vi "Vision Center Shoot.vi"(0 "Intake":dbl=1.0, 1 "X axis value":dbl=0.05 format="%#_13g", 2 "X axis value 2":dbl=-0.05) -> ()   [LabVIEW 2015]
uses:
  Robot Global Data.vi
panel:
  in  "X axis value 3":dbl=0.05 format="%#_13g"
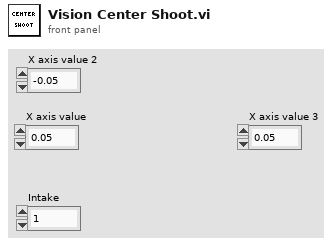
[diagram p1: front panel]
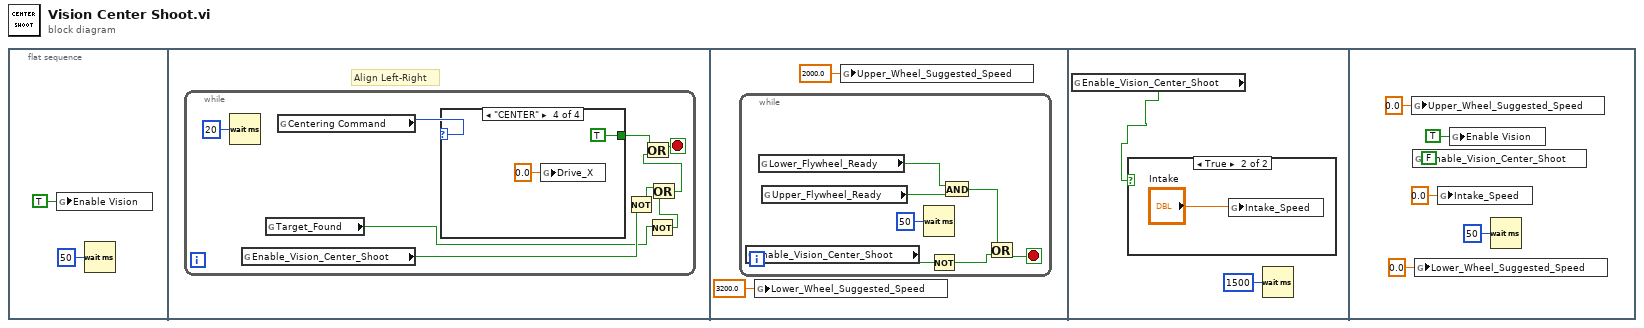
[diagram p0: block diagram]
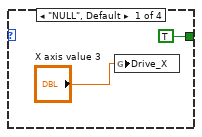
[diagram p2: hidden frame]
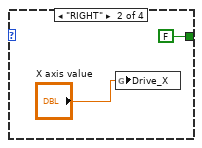
[diagram p3: hidden frame]
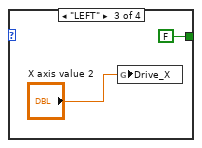
[diagram p4: hidden frame]
diagram:
  n1 = flat-sequence {
    frame #0 {
      n2 = global write "Robot Global Data.vi" "Enable Vision"(TRUE ("Enable Vision")) -> ()
      n3 = Wait (ms)(milliseconds to wait=u32 50) -> ()  [unwired: 1 out]
    }
    frame #1 {
      # "Align Left-Right"
      n4 = while {
        stop <- w8 stop-if-true
        n5 = Wait (ms)(milliseconds to wait=u32 20) -> ()  [unwired: 1 out]
        n6 = global read "Robot Global Data.vi" "Enable_Vision_Center_Shoot"() -> (w7:bool)
        n7 = global read "Robot Global Data.vi" "Target_Found"() -> (w5:bool)
        n8 = global read "Robot Global Data.vi" "Centering Command"() -> (w10:enum16{"NULL", "RIGHT", "LEFT", "CENTER"})
        n9 = case shown="\"CENTER\"" w10 {
          tunnel: [TRUE FALSE FALSE TRUE] -> w11
          frame "NULL", Default {
            n10 = global write "Robot Global Data.vi" "Drive_X"("X axis value 3") -> ()
          }
          frame "RIGHT" {
            n11 = global write "Robot Global Data.vi" "Drive_X"("X axis value") -> ()
          }
          frame "LEFT" {
            n12 = global write "Robot Global Data.vi" "Drive_X"("X axis value 2") -> ()
          }
          frame "CENTER" {
            n13 = global write "Robot Global Data.vi" "Drive_X"(0.0 ("Drive_X")) -> ()
          }
        }
        n14 = Not(x=w7) -> (.not. x?=w6:bool)
        n15 = Not(x=w5) -> (.not. x?=w4:bool)
        n16 = Or(x=w6, y=w4) -> (x .or. y?=w3:bool)
        n17 = Or(x=w11, y=w3) -> (x .or. y?=w8:bool)
      }
    }
    frame #2 {
      n18 = while {
        stop <- w24 stop-if-true
        n19 = global read "Robot Global Data.vi" "Enable_Vision_Center_Shoot"() -> (w23:bool)
        n20 = global read "Robot Global Data.vi" "Lower_Flywheel_Ready"() -> (w27:bool)
        n21 = global read "Robot Global Data.vi" "Upper_Flywheel_Ready"() -> (w28:bool)
        n22 = Wait (ms)(milliseconds to wait=u32 50) -> ()  [unwired: 1 out]
        n23 = Not(x=w23) -> (.not. x?=w22:bool)
        n24 = And(x=w27, y=w28) -> (x .and. y?=w26:bool)
        n25 = Or(x=w26, y=w22) -> (x .or. y?=w24:bool)
      }
      n26 = global write "Robot Global Data.vi" "Lower_Wheel_Suggested_Speed"(3200.0 ("Lower_Wheel_Suggested_Speed")) -> ()
      n27 = global write "Robot Global Data.vi" "Upper_Wheel_Suggested_Speed"(2000.0 ("Upper_Wheel_Suggested_Speed")) -> ()
    }
    frame #3 {
      n28 = global read "Robot Global Data.vi" "Enable_Vision_Center_Shoot"() -> (w29:bool)
      n29 = case shown="True" w29 {
        frame False {
        }
        frame True {
          n30 = global write "Robot Global Data.vi" "Intake_Speed"("Intake") -> ()
        }
      }
      n31 = Wait (ms)(milliseconds to wait=u32 1500) -> ()  [unwired: 1 out]
    }
    frame #4 {
      n32 = global write "Robot Global Data.vi" "Upper_Wheel_Suggested_Speed"(0.0 ("Upper_Wheel_Suggested_Speed")) -> ()
      n33 = global write "Robot Global Data.vi" "Enable_Vision_Center_Shoot"(FALSE ("Enable_Shooter")) -> ()
      n34 = global write "Robot Global Data.vi" "Lower_Wheel_Suggested_Speed"(0.0 ("Lower_Wheel_Suggested_Speed")) -> ()
      n35 = global write "Robot Global Data.vi" "Intake_Speed"(0.0 ("Intake_Speed")) -> ()
      n36 = global write "Robot Global Data.vi" "Enable Vision"(TRUE ("Enable Vision")) -> ()
      n37 = Wait (ms)(milliseconds to wait=u32 50) -> ()  [unwired: 1 out]
    }
  }
